vi "ScanDelay_FTIR_AcquireInterferogram.vi"(9 "Sampling rate":dbl=250000.0, 10 "Time per acquisiton (s)":dbl=0.125) -> (3 "Output V-d array":dbl[][](array[numeric]))   [LabVIEW 2021]
panel:
  in  "Plot?":bool
  out "Acquisition cycle":dbl[][](graph)
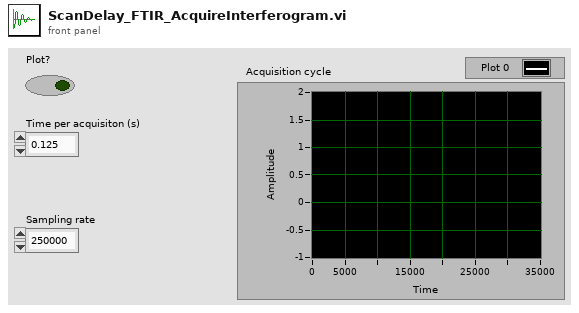
[diagram p1: front panel]
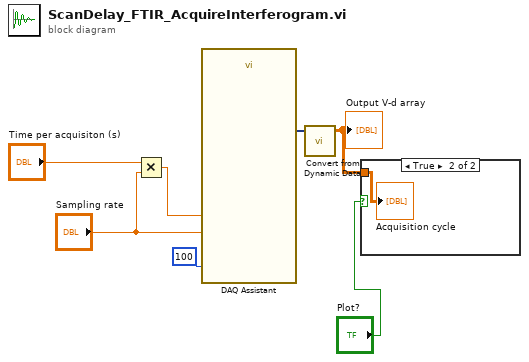
[diagram p0: block diagram]
diagram:
  n1 = Multiply(x="Time per acquisiton (s)", y="Sampling rate") -> (x*y=w6:dbl)
  n2 = call "DAQ Assistant"("rate"="Sampling rate", "number of samples"=w6, "timeout (s)"=100) -> ("data"=w7:dynamicdata)  [unwired: 14 in, 2 out]
  n3 = call "Convert from Dynamic Data"("Dynamic Data Type"=w7) -> ("Array"=w2:dbl[][])  [unwired: 3 in]
  "Output V-d array" <- w2
  n4 = case shown="True" "Plot?" {
    tunnel: w2 -> [_ w8]
    frame False {
    }
    frame True {
      "Acquisition cycle" <- w8
    }
  }
